vi "InitCSMs.vi"(8 "error in":errorcluster, 11 "testcase-CSMArgument.lvclass in":refnum<class "testcase-CSMArgument.lvclass">) -> (0 "error out":errorcluster, 3 "testcase-CSMArgument.lvclass out":refnum<class "testcase-CSMArgument.lvclass">)   [LabVIEW 2017, in "testcase-CSMArgument.lvclass"]
uses:
  testcase-CSMArgument.lvclass
  testcase-CSMArgument.lvclass/testcase-CSMArgument.ctl
  CSM/Normal-CSM.vi
  src/user.lib/_NEVSTOP/Communicable State Machine(CSM)/Communicable State Machine.lvlib
  CSM/CSM-Testcase.lvlib
panel:
  out "Waited (ms)":u32
  out "CSMs Left":string[](array[string])
  out "CSMs":string[](array[string])
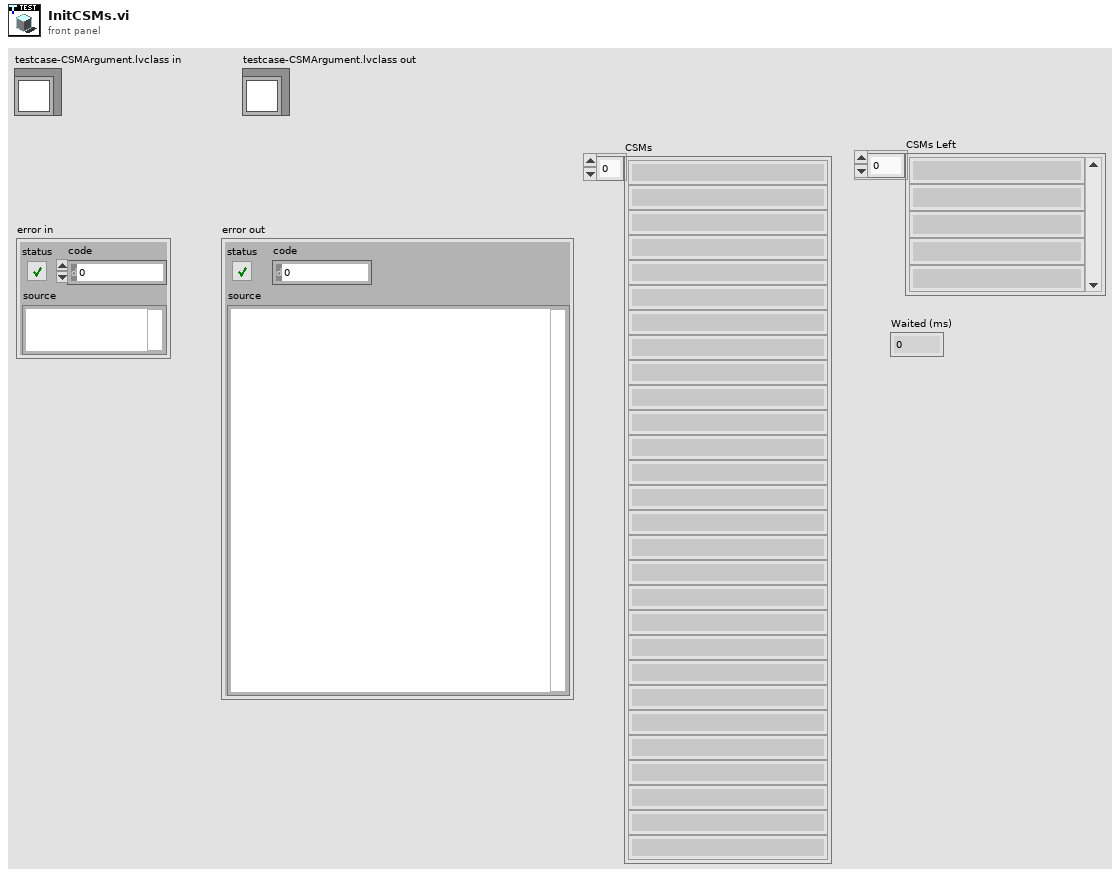
[diagram p1: front panel]
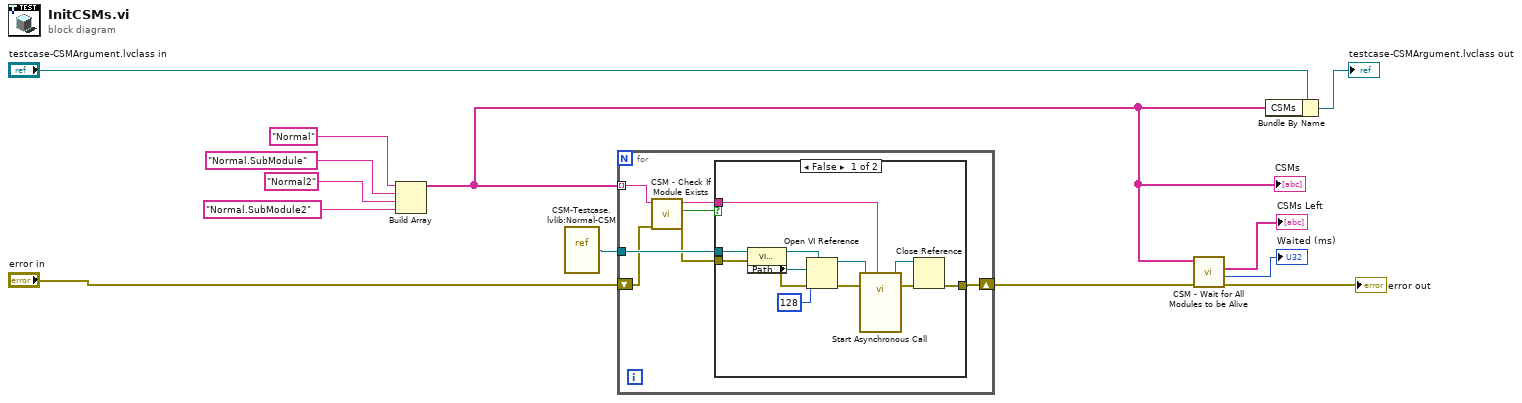
[diagram p0: block diagram]
diagram:
  n1 = Build Array("Normal" ("Name (\"\" to Use UUID)"), "Normal.SubModule" ("Name (\"\" to Use UUID)"), "Normal2" ("Name (\"\" to Use UUID)"), "Normal.SubModule2" ("Name (\"\" to Use UUID)")) -> (w3:string[])
  "CSMs" <- w3
  n2 = vi-ref "CSM-Testcase.lvlib:Normal-CSM.vi"() -> (w10:refnum<vi>)
  n3 = for {
    tunnel: w10 -> [w20]
    tunnel: w3 -> [w17] mode=indexing
    shift-right: [w14] -> w5
    shift-left: "error in" -> [w19]
    n4 = call "CSM - Check If Module Exists.vi"("Error In"=w19, "CSM Name"=w17) -> ("error out"=w18:errorcluster, "Exist?"=w15:bool, "CSM Name (Dup)"=w16:string)  [unwired: 7 in]
    n5 = case shown="False" w15 {
      tunnel: w20 -> [w24 _]
      tunnel: [w23 w33] -> w14
      tunnel: w18 -> [w22 w33]
      tunnel: w16 -> [w21 _]
      frame False {
        n6 = property class="VI (strict)"(reference=w24, error in=w22) -> (reference out=w30:refnum<vi>, error out=w28:errorcluster, "Path"=w27:path)
        n7 = Open VI Reference(type specifier VI Refnum (for type only)=w30, vi path=w27, options=128, error in (no error)=w28) -> (vi reference=w26:refnum<vi>, error out=w31:errorcluster)  [unwired: 2 in]
        n8 = call-by-ref "Start Asynchronous Call"(reference=w26, error in=w31, "Name (\"\" to Use UUID)"=w21) -> (reference out=w25:refnum<vi>, error out=w29:errorcluster)  [unwired: 11 in]
        n9 = Close Reference(reference=w25, error in (no error)=w29) -> (error out=w23:errorcluster)
      }
      frame True {
      }
    }
  }
  n10 = call "CSM - Wait for All Modules to be Alive.vi"("Error In"=w5, "CSM Names"=w3) -> ("error out"=→"error out":errorcluster, "Waited (ms)"=→"Waited (ms)":u32, "CSMs Left"=→"CSMs Left":string[])  [unwired: 7 in]
  n11 = Bundle By Name(cluster="testcase-CSMArgument.lvclass in", "CSMs"=w3) -> (→"testcase-CSMArgument.lvclass out":refnum<class "testcase-CSMArgument.lvclass">)
